vi "SeCrTs-Unbalanced Protection.vi"(8 "Common Threshold":dbl, 9 "RMS Ic":dbl[](array[numeric]), 10 "RMS Ib":dbl[](array[numeric]), 11 "RMS Ia":dbl[](array[numeric])) -> (0 "Overall":bool)   [LabVIEW 2022 SP3]
panel:
  out "Ic Un":bool
  out "Ib Un":bool
  out "Ia Un":bool
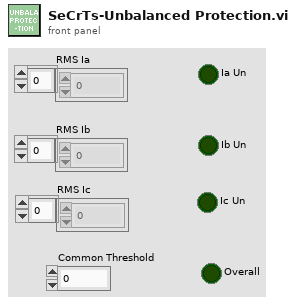
[diagram p1: front panel]
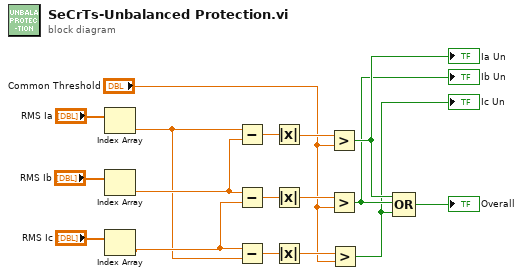
[diagram p0: block diagram]
diagram:
  n1 = Index Array(array="RMS Ia") -> (element=w12:dbl)  [unwired: 1 in]
  n2 = Index Array(array="RMS Ib") -> (element=w14:dbl)  [unwired: 1 in]
  n3 = Index Array(array="RMS Ic") -> (element=w13:dbl)  [unwired: 1 in]
  n4 = Subtract(x=w12, y=w14) -> (x-y=w11:dbl)
  n5 = Subtract(x=w14, y=w13) -> (x-y=w10:dbl)
  n6 = Subtract(x=w13, y=w12) -> (x-y=w9:dbl)
  n7 = Absolute Value(x=w11) -> (abs(x)=w8:dbl)
  n8 = Absolute Value(x=w10) -> (abs(x)=w7:dbl)
  n9 = Absolute Value(x=w9) -> (abs(x)=w6:dbl)
  n10 = Greater?(x=w8, y="Common Threshold") -> (0:w5:bool)
  "Ia Un" <- w5
  n11 = Greater?(x=w7, y="Common Threshold") -> (0:w3:bool)
  "Ib Un" <- w3
  n12 = Greater?(x=w6, y="Common Threshold") -> (0:w2:bool)
  "Ic Un" <- w2
  n13 = Compound Arithmetic op=OR(w5, w3, w2) -> (→"Overall":bool)
